vi "CaptureSnapshot.vi"(0 "object in":refnum<class "Hamamatsu.lvclass">, 2 "Timeout":i32=-1, 5 "error in (no error)":errorcluster) -> (14 "object out":refnum<class "Hamamatsu.lvclass">, 16 "FreeRunningImage":T1, 17 "Timestamp":dbl, 19 "error out":errorcluster)   [LabVIEW 2024, in "Hamamatsu.lvclass"]
uses:
  Hamamatsu.lvclass
  <vilib>/vision/Image Controls.llb/IMAQ Image.ctl
  Hamamatsu.lvclass/Hamamatsu.ctl
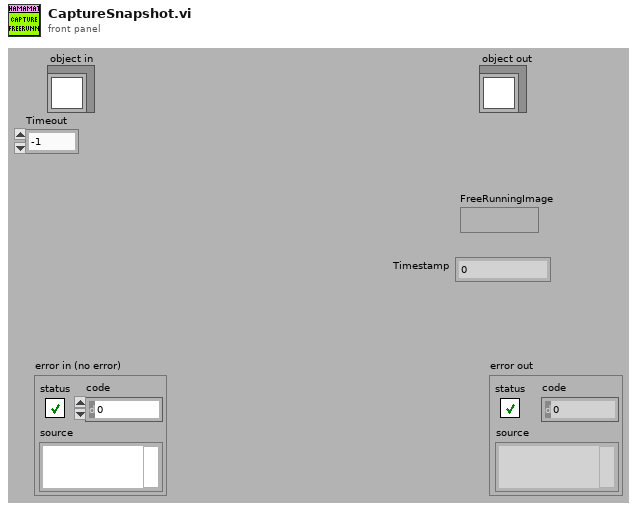
[diagram p1: front panel]
types:
  T1 = typedef "IMAQ Image.ctl" = refnum<image>
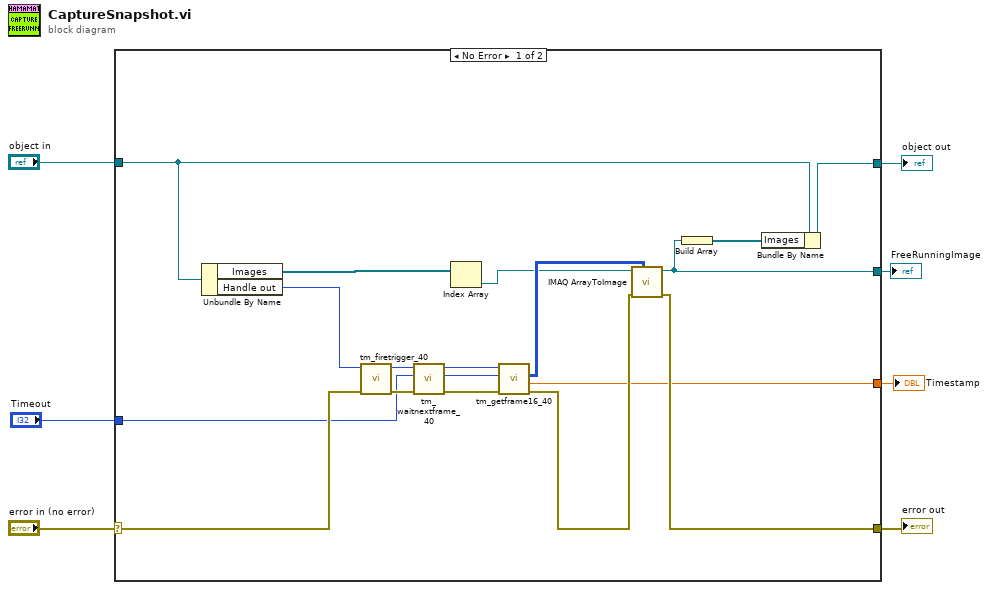
[diagram p0: block diagram]
diagram:
  n1 = case shown="No Error" "error in (no error)" {
    selector: "error in (no error)" -> [w10 w27]
    tunnel: [w19 w27] -> w6
    tunnel: [w24 w26] -> w4
    tunnel: "object in" -> [w25 w26]
    tunnel: [w14 _] -> w3
    tunnel: [w13 _] -> w2
    tunnel: "Timeout" -> [w8 _]
    frame No Error {
      n2 = Unbundle By Name(w25) -> ("Images"=w17:T1[], "Handle out"=w12:u32)
      n3 = call <userlib>:"tm_firetrigger_40.vi"("error in (no error)"=w10, "Handle in"=w12) -> ("error out"=w9:errorcluster, "Handle out"=w11:u32)  [unwired: 8 in]
      n4 = call <userlib>:"tm_waitnextframe_40.vi"("error in (no error)"=w9, "Timeout"=w8, "Handle in"=w11) -> ("error out"=w22:errorcluster, "Frame Index"=w18:i32, "Handle out"=w23:u32)  [unwired: 5 in, 1 out]
      n5 = Index Array(array=w17) -> (element=w16:T1)  [unwired: 1 in]
      n6 = call <userlib>:"tm_getframe16_40.vi"("error in (no error)"=w22, "Frame Index"=w18, "Handle in"=w23) -> ("error out"=w20:errorcluster, "Timestamp"=w13:dbl, "Data"=w21:u16[][])  [unwired: 5 in, 1 out]
      n7 = call "IMAQ ArrayToImage"("Image Pixels (U16)"=w21, "error in (no error)"=w20, "Image"=w16) -> ("error out"=w19:errorcluster, "Image Out"=w14:T1)  [unwired: 7 in]
      n8 = Build Array(w14) -> (w15:T1[])
      n9 = Bundle By Name(cluster=w25, "Images"=w15) -> (w24:refnum<class "Hamamatsu.lvclass">)
    }
    frame Error {
    }
  }
  "error out" <- w6
  "object out" <- w4
  "FreeRunningImage" <- w3
  "Timestamp" <- w2
